vi "Heating or cooling global.vi"() -> ()   [LabVIEW 2015]
panel:
  out "heating or cooling":string
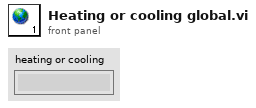
[diagram p1: front panel]
diagram:
